vi "Fetch.vi"   [LabVIEW 2011, in "Agilent 34401.lvlib"]
doc: "This low level VI fetches and returns measurements.\n\n<B>Note:</B>\n\nThis VI has been obsoleted from the driver and is included for compatibility with existing applications. New applications should use the <B>Fetch Measurement VI</B>."
uses:
  <instrlib>/Agilent 34401/Agilent 34401.lvlib
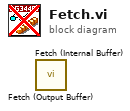
[diagram p0: block diagram]
diagram:
  n1 = call <instrlib>:"Fetch (Output Buffer).vi"() -> ()  [unwired: 8 in, 4 out]
  n2 = call <instrlib>:"Fetch (Internal Buffer).vi"() -> ()  [unwired: 9 in, 3 out]
